vi "Post-Build Action_AddToIni_DefaultFont.vi"(5 "Files Generated by Build":path[](array[path]) caption="ビルドで生成されたファイル", 6 "Top Level/Always Included VIs":path[](array[path]) caption="トップレベル/常に含むVI", 7 "Destination Path":path caption="出力先パス", 8 "error in (no error)":errorcluster caption="エラー入力（エラーなし）", 9 "Target Name":string caption="ターゲット名", 10 "Build Specification Name":string caption="ビルド仕様名", 11 "Project Path":path caption="プロジェクトパス") -> (0 "error out":errorcluster caption="エラー出力")   [LabVIEW 2009]
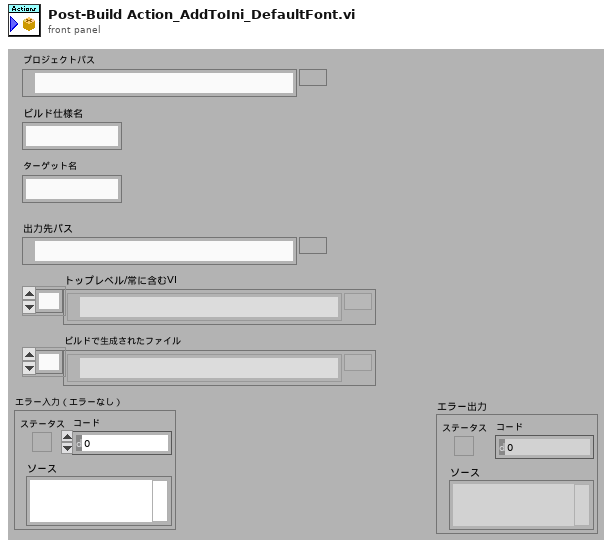
[diagram p1: front panel]
types:
  T1 = enum16{"open", "replace", "create", "open or create", "replace or create", "replace or create with confirmation"}
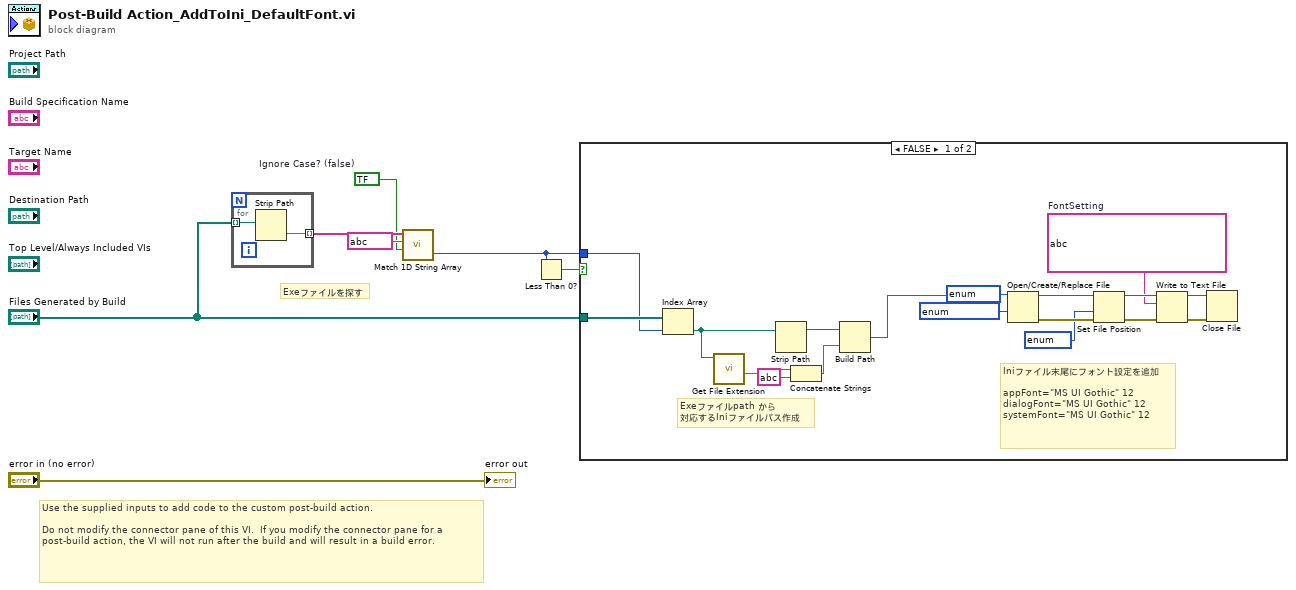
[diagram p0: block diagram]
diagram:
  w3 = bool ?  # Ignore Case? (false)
  # "Exeファイルを探す"
  # "Use the supplied inputs to add code to the custom post-build action.\n\nDo not modify the connector pane of this VI.  If you modify the connector pane for a post-build action, the VI will not run after the build and will result in a build error."
  n1 = for {
    tunnel: "Files Generated by Build" -> [w9] mode=indexing
    tunnel: [w8] -> w5 mode=indexing
    n2 = Strip Path(path=w9) -> (name=w8:string)  [unwired: 1 out]
  }
  n3 = call <vilib>:"Match 1D String Array.vi"("Ignore Case? (false)"=w3, "Pattern"=string ?, "Strings"=w5) -> ("index of element"=w1:i32)  [unwired: 1 in, 1 out]
  n4 = Less Than 0?(x=w1) -> (x < 0?=w2:bool)
  n5 = case shown="FALSE" w2 {
    tunnel: "Files Generated by Build" -> [w17 _]
    tunnel: w1 -> [w16 _]
    frame #0 {
      w18 = string ?  # FontSetting
      # "Iniファイル末尾にフォント設定を追加\n\nappFont=\"MS UI Gothic\" 12\ndialogFont=\"MS UI Gothic\" 12\nsystemFont=\"MS UI Gothic\" 12"
      # "Exeファイルpath から\n対応するIniファイルパス作成"
      n6 = Index Array(array=w17, index=w16) -> (element=w15:path)
      n7 = call <vilib>:"Get File Extension.vi"("file"=w15) -> ("filename without extension"=w14:string)  [unwired: 7 in, 3 out]
      n8 = Strip Path(path=w15) -> (stripped path=w12:path)  [unwired: 1 out]
      n9 = Concatenate Strings(w14, string ? ("文字列")) -> (w11:string)
      n10 = Build Path(base path=w12, name or relative path=w11) -> (appended path=w10:path)
      n11 = Open/Create/Replace File(file path (use dialog)=w10, operation (0:open)=T1 ? ("操作（0:open）"), access (0:read/write)=enum16{"read/write", "read-only", "write-only"} ? ("アクセス （0:read/write）")) -> (refnum out=w26:refnum<file>, error out=w25:errorcluster)  [unwired: 3 in, 1 out]
      n12 = Set File Position(refnum=w26, from (0:start)=enum16{"start", "end", "current"} ? ("基点（0:start）")) -> (refnum out=w20:refnum<file>)  [unwired: 2 in, 1 out]
      n13 = Write to Text File(file (use dialog)=w20, text=w18, error in=w25) -> (refnum out=w22:refnum<file>, error out=w21:errorcluster)  [unwired: 1 in, 1 out]
      n14 = Close File(refnum=w22, error in=w21) -> ()  [unwired: 2 out]
    }
    frame #1 {
      # "Exeが見つからない"
    }
  }
  "error out" <- "error in (no error)"
